vi "create status logfile line (subVI).vi"(9 "cam status":bool, 10 "2p status":bool, 11 "relative seconds":dbl) -> (2 "string []":string[](array[string]))   [LabVIEW 2021]
uses:
  global-variables/global variables.vi
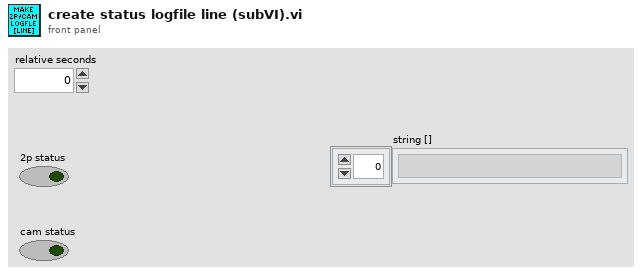
[diagram p1: front panel]
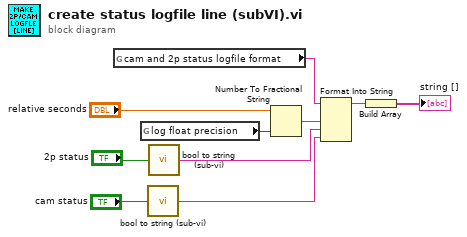
[diagram p0: block diagram]
diagram:
  n1 = global read "global variables.vi" "cam and 2p status logfile format"() -> (w9:string)
  n2 = global read "global variables.vi" "log float precision"() -> (w8:i16)
  n3 = call "bool to string (sub-vi).vi"("Boolean"="cam status") -> ("String"=w1:string)
  n4 = call "bool to string (sub-vi).vi"("Boolean"="2p status") -> ("String"=w2:string)
  n5 = Number To Fractional String(number="relative seconds", precision (6)=w8) -> (F-format string=w6:string)  [unwired: 2 in]
  n6 = Format Into String(format string=w9, w6, w2, w1) -> (resulting string=w7:string)  [unwired: 2 in, 1 out]
  n7 = Build Array(w7) -> (→"string []":string[])
